vi "Update Total Duration.vi"(8 "error in (no error)":errorcluster, 9 "Free Run?":bool, 10 "# Repeats":u16, 11 "User Interface in":refnum<class "User Interface.lvclass">) -> (0 "error out":errorcluster, 3 "User Interface out":refnum<class "User Interface.lvclass">)   [LabVIEW 2016, in "_User Interface.lvlib" / "User Interface.lvclass"]
uses:
  User Interface.lvclass
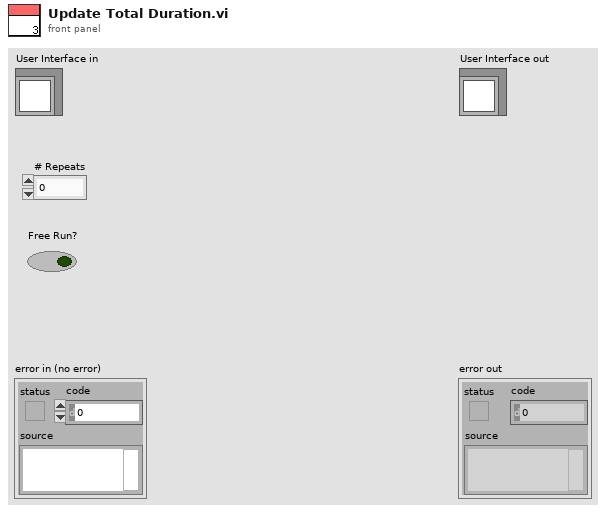
[diagram p1: front panel]
types:
  T1 = enum8{"Enabled", "Disabled", "Disabled and Grayed Out"}
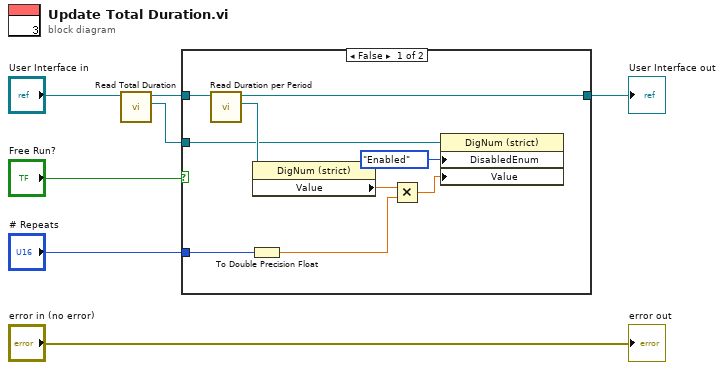
[diagram p0: block diagram]
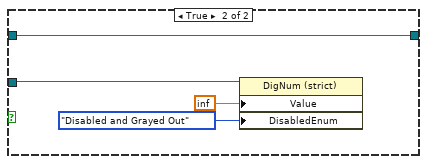
[diagram p2: hidden frame]
diagram:
  n1 = call-dynamic "Read Total Duration.vi"("User Interface in"="User Interface in") -> ("Total Duration"=w7:refnum<vi>, "User Interface out"=w2:refnum<class "User Interface.lvclass">)  [unwired: 9 in]
  n2 = case shown="False" "Free Run?" {
    tunnel: w7 -> [w12 w20]
    tunnel: [w14 w18] -> w3
    tunnel: w2 -> [w16 w18]
    tunnel: "# Repeats" -> [w11 _]
    frame False {
      n3 = call-dynamic "Read Duration per Period.vi"("User Interface in"=w16) -> ("Duration per Period"=w15:refnum<vi>, "User Interface out"=w14:refnum<class "User Interface.lvclass">)  [unwired: 9 in]
      n4 = To Double Precision Float(number=w11) -> (double precision float=w10:dbl)
      n5 = property class="DigNum (strict)"(reference=w15) -> ("Value"=w13:dbl)  [unwired: 1 in, 2 out]
      n6 = Multiply(x=w13, y=w10) -> (x*y=w9:dbl)
      n7 = property class="DigNum (strict)"(reference=w12, "DisabledEnum"=T1."Enabled" ("Disabled"), "Value"=w9) -> ()  [unwired: 1 in, 2 out]
    }
    frame True {
      n8 = property class="DigNum (strict)"(reference=w20, "Value"=inf, "DisabledEnum"=T1."Disabled and Grayed Out" ("Disabled")) -> ()  [unwired: 1 in, 2 out]
    }
  }
  "User Interface out" <- w3
  "error out" <- "error in (no error)"
